vi "Process File.vi"(8 "error in (no error)":errorcluster, 10 "File":refnum<class "Acquired Result.lvclass">, 11 "Line Detector in":refnum<class "Resonance Detector.lvclass">) -> (0 "error out":errorcluster, 2 "File out":refnum<class "Acquired Result.lvclass">, 3 "Line Detector out":refnum<class "Resonance Detector.lvclass">)   [LabVIEW 2016, in "Resonance Detector.lvclass"]
uses:
  Resonance Detector.lvclass
  NHMFL_Core/Libraries/Instruments/Results/Acquired Result/Acquired Result.lvclass
  Read Line detector configuration.vi
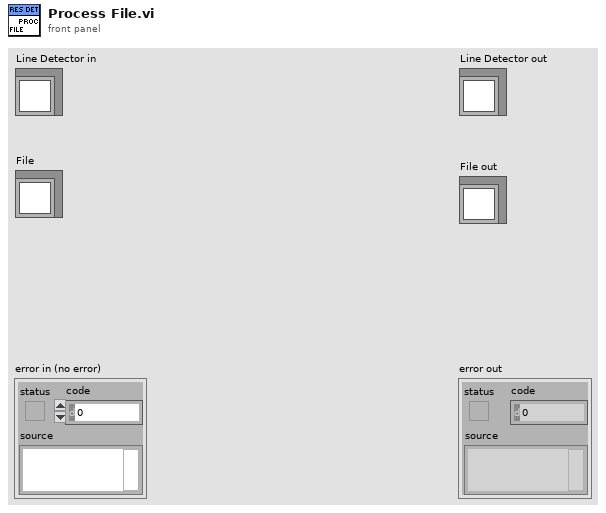
[diagram p1: front panel]
types:
  T1 = typedef "Line Detector Configuration.ctl" = cluster{"Peak width guess":dbl, "Background removal":enum16{"NONE", "High-pass", "Detrend"}, "Smoothing":enum16{"NONE", "Low-pass", "Denoise"}, "Smooth window":dbl, "Relative threshold":dbl, "Finder algorithm":enum16{"Basic", "Wavelet", "Wavelet+detrend"}, "Bgd window":dbl, "Spectrum recorder module name":string, "Fit window":dbl, "Initial fit guess":enum16{"Peak finder", "Last fit"}, "Follow\npeaks":bool, "Re-sample":dbl}
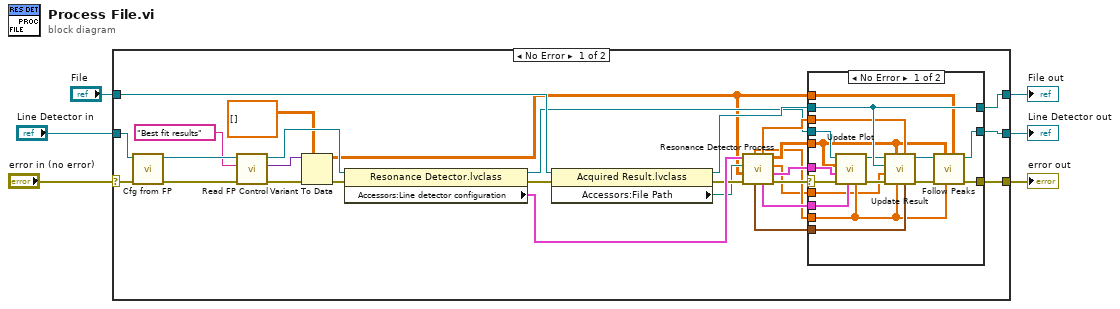
[diagram p0: block diagram]
diagram:
  n1 = case shown="No Error" "error in (no error)" {
    selector: "error in (no error)" -> [w33 w56]
    tunnel: "Line Detector in" -> [w34 w57]
    tunnel: "File" -> [w19 w58]
    tunnel: [w32 w58] -> w3
    tunnel: [w15 w57] -> w2
    tunnel: [w16 w56] -> w1
    frame No Error {
      n2 = call-dynamic "Cfg from FP.vi"("error in (no error)"=w33, "Measure Object in"=w34) -> ("error out"=w25:errorcluster, "Measure Object out"=w27:refnum<class "Resonance Detector.lvclass">)  [unwired: 8 in]
      n3 = call-dynamic "Read FP Control.vi"("error in (no error)"=w25, "Control Name"="Best fit results", "Measure Object in"=w27) -> ("error out"=w23:errorcluster, "Control Value"=w22:variant, "Measure Object out"=w26:refnum<class "Resonance Detector.lvclass">)  [unwired: 5 in, 1 out]
      n4 = Variant To Data(error in=w23, type=dbl[][] [] ("Best fit results"), Variant=w22) -> (data=w8:dbl[][], error out=w21:errorcluster)
      n5 = property class="Resonance Detector.lvclass"(reference=w26, error in=w21) -> (reference out=w13:refnum<class "Resonance Detector.lvclass">, error out=w18:errorcluster, "Accessors:Line detector configuration"=w28:T1)
      n6 = property class="Acquired Result.lvclass"(reference=w19, error in=w18) -> (reference out=w17:refnum<class "Acquired Result.lvclass">, error out=w14:errorcluster, "Accessors:File Path"=w11:path)
      n7 = call "Resonance Detector Process.vi"("error in (no error)"=w14, "Best fit guess"=w8, "File"=w11, "Line Detector Configuration"=w28) -> ("error out"=w12:errorcluster, "Plots"=w35:cluster{"X":dbl[], "Array":dbl[]}[], "Peaks absolute time"=w7:dbl[], "Best fit results"=w30:dbl[][], "Peak Plot"=w10:cluster{"Ramp Pattern":dbl[], "X":dbl[]}[], "Peaks"=w31:dbl[], "sp time"=w29:timestamp, "Good fit?"=w9:dbl[])
      n8 = case shown="No Error" w12 {
        selector: w12 -> [w50 w55]
        tunnel: w35 -> [w52 _]
        tunnel: [w48 w53] -> w32
        tunnel: w31 -> [w47 _]
        tunnel: w30 -> [w43 _]
        tunnel: w29 -> [w46 _]
        tunnel: w17 -> [w48 w53]
        tunnel: [w37 w55] -> w16
        tunnel: [w39 w54] -> w15
        tunnel: w13 -> [w49 w54]
        tunnel: w10 -> [w51 _]
        tunnel: w9 -> [w41 _]
        tunnel: w8 -> [w42 _]
        tunnel: w7 -> [w36 _]
        frame No Error {
          n9 = call-dynamic "Update Plot.vi"("Good fit?"=w41, "Peak Plot"=w51, "error in (no error)"=w50, "Plots"=w52, "Best fit results"=w43, "Resonance Detector in"=w49) -> ("error out"=w38:errorcluster, "Resonance Detector out"=w40:refnum<class "Resonance Detector.lvclass">)  [unwired: 4 in]
          n10 = call-dynamic "Update Result.vi"("sp time stamp"=w46, "Peaks"=w47, "Good fit?"=w41, "Best fit results"=w43, "error in (no error)"=w38, "Peaks absolute time"=w36, "File"=w48, "Resonance Detector in"=w40) -> ("error out"=w44:errorcluster, "Resonance Detector out"=w45:refnum<class "Resonance Detector.lvclass">)  [unwired: 1 in, 1 out]
          n11 = call-dynamic "Follow Peaks.vi"("Best fit guess"=w42, "Good fit?"=w41, "Best fit results"=w43, "error in (no error)"=w44, "Resonance Detector in"=w45) -> ("error out"=w37:errorcluster, "Resonance Detector out"=w39:refnum<class "Resonance Detector.lvclass">)  [unwired: 5 in]
        }
        frame Error {
        }
      }
    }
    frame Error {
    }
  }
  "error out" <- w1
  "Line Detector out" <- w2
  "File out" <- w3
